vi "CTRE_PigeonIMU_SetStatusFrameRate.vi"(8 "error in (no error)":errorcluster, 9 "StatusFrame":T1 items=["CondStatus_1_General"=2, "CondStatus_9_SixDeg_YPR"=3, "CondStatus_6_SensorFusion"=4, "CondStatus_11_GyroAccum"=5, "CondStatus_2_GeneralCompass"=11, "CondStatus_3_GeneralAccel"=12, "CondStatus_10_SixDeg_Quat"=14, "RawStatus_4_Mag"=6, "BiasedStatus_2_Gyro"=8, "BiasedStatus_4_Mag"=9, "BiasedStatus_6_Accel"=10], 10 "Period (ms)":i16, 11 "PigeonIMUDevRef":T2={"DeviceStatus"={"status"=FALSE, "code"=0, "source"=""}, "Device Number"=0, "Type"=352321536, "Device ID"=0} {"Type" items=["CAN"=352321536, "TalonSRX"=33554432]}) -> (0 "error out":errorcluster, 3 "PigeonIMUDevRef":T2={"DeviceStatus"={"status"=FALSE, "code"=0, "source"=""}, "Device Number"=0, "Type"=352321536, "Device ID"=0} {"Type" items=["CAN"=352321536, "TalonSRX"=33554432]})   [LabVIEW 2016]
doc: "Period (ms) sets the rate at which StatusFrame is sent."
uses:
  <vilib>/Rock Robotics/WPI/ThirdParty/Sensors/Pigeon IMU/CTRE_PigeonIMU_DeviceRef.ctl
  <vilib>/Rock Robotics/WPI/ThirdParty/Sensors/Pigeon IMU/CTRE_PigeonIMU_ConnectionType.ctl
  <vilib>/Rock Robotics/WPI/ThirdParty/Sensors/Pigeon IMU/CTRE_PigeonIMU_StatusFrameRate.ctl
  <vilib>/Rock Robotics/WPI/ThirdParty/Sensors/Pigeon IMU/CTRE_PigeonIMU_Params.ctl
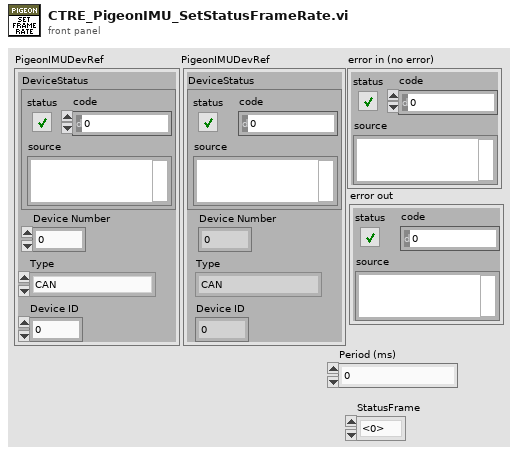
[diagram p1: front panel]
types:
  T1 = typedef "CTRE_PigeonIMU_StatusFrameRate.ctl" = u16
  T2 = typedef "CTRE_PigeonIMU_DeviceRef.ctl" = cluster{"DeviceStatus":errorcluster, "Device Number":u8, "Type":T3, "Device ID":u32}
  T3 = typedef "CTRE_PigeonIMU_ConnectionType.ctl" = u32
  T4 = typedef "CTRE_PigeonIMU_Params.ctl" = u8
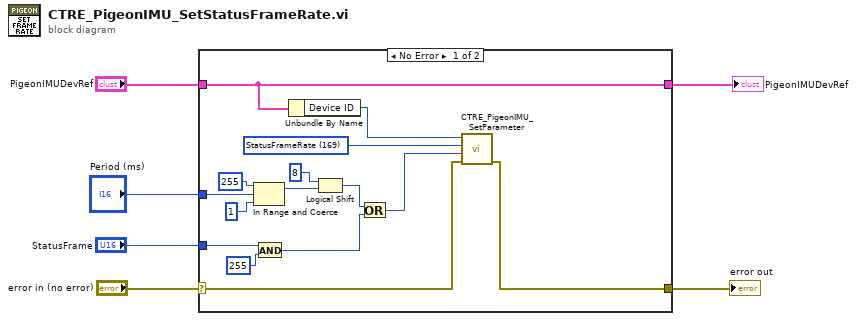
[diagram p0: block diagram]
diagram:
  n1 = case shown="No Error" "error in (no error)" {
    selector: "error in (no error)" -> [w19 w22]
    tunnel: [w18 w22] -> w5
    tunnel: [w21 w23] -> w3
    tunnel: "PigeonIMUDevRef" -> [w21 w23]
    tunnel: "Period (ms)" -> [w16 _]
    tunnel: "StatusFrame" -> [w13 _]
    frame No Error {
      w17 = T4 169 items=["YawOffset"=160, "CompassOffset"=161, "BetaGain"=162, "Reserved163"=163, "GyroNoMotionCal"=164, "EnterCalibration"=165, "FusedHeadingOffset"=166, "StatusFrameRate"=169, "AccumZ"=170, "TempCompDisable"=171] ("Parameter")
      n2 = In Range and Coerce(upper limit=i16 255, x=w16, lower limit=i16 1) -> (coerced(x)=w11:i16)  [unwired: 1 out]
      n3 = And(x=w13, y=u16 255 ("upper limit")) -> (x .and. y?=w8:T1)
      n4 = Unbundle By Name(w21) -> ("Device ID"=w20:u32)
      n5 = Logical Shift(y=i16 8, x=w11) -> (x << y=w9:i16)
      n6 = Or(x=w9, y=w8) -> (x .or. y?=w7:T1)
      n7 = call <vilib>:"CTRE_PigeonIMU_SetParameter.vi"("error in (no error)"=w19, "Value"=w7, "Parameter"=w17, "Device ID (0)"=w20) -> ("error out"=w18:errorcluster)  [unwired: 6 in, 1 out]
    }
    frame Error {
    }
  }
  "PigeonIMUDevRef" <- w3
  "error out" <- w5
